vi "prompts get.vi"(8 "error in":errorcluster, 10 "id":i32, 11 "message json":string) -> (0 "error out":errorcluster, 3 "response":string)   [LabVIEW 2020, in "MCP Server.lvlib"]
uses:
  MCP Server.lvlib
  Output Parameter.ctl
  Input Parameter.ctl
  36169f03-25f9-42a4-b558-7da57aa14dd0.vi
  7d3bd472-2036-4192-96a4-2be547f36210.vi
  14c59c94-2525-420a-b2b2-c4c9036dcf4d.vi
  <vilib>/JDP Science/JSONtext/Next JSON Value.vi
  <vilib>/JDP Science/JSONtext/String Subset.vi
  <vilib>/JDP Science/JSONtext/Parsing/Advance past next JSON Value (inlined COPY).vi
  <vilib>/JDP Science/JSONtext/Parsing/Advance past whitespace.vi
  <vilib>/JDP Science/JSONtext/Parsing/Advance past String.vi
  <vilib>/JDP Science/JSONtext/Parsing/Advance past Number.vi
  <vilib>/JDP Science/JSONtext/Parsing/Advance past Line Ending.vi
  <vilib>/JDP Science/JSONtext/Parsing/Parse Full Path or Item Name.vi
  <vilib>/JDP Science/JSONtext/Parsing/Advance past Array.vi
  <vilib>/JDP Science/JSONtext/Parsing/Advance past Object.vi
  <vilib>/JDP Science/JSONtext/support/Error Cluster From Code.vi
  <vilib>/JDP Science/JSONtext/Offset/Find Item Locations by Path.vi
  <vilib>/JDP Science/JSONtext/JSON text to Variant.vi
  <vilib>/Utility/error.llb/Error Cluster From Error Code.vi
  <vilib>/JDP Science/JSONtext/Variant to JSON Text.vi
  <vilib>/JDP Science/JSONtext/support/Format JSON Object.vi
  <vilib>/JDP Science/JSONtext/support/Format JSON Array Text.vi
  <vilib>/JDP Science/JSONtext/LVClass Serializer/JSONtext LVClass Serializer.lvclass
  <vilib>/ErrorRing/Error Ring.xnode
  <vilib>/JDP Science/JSONtext/JSONtext.lvlib
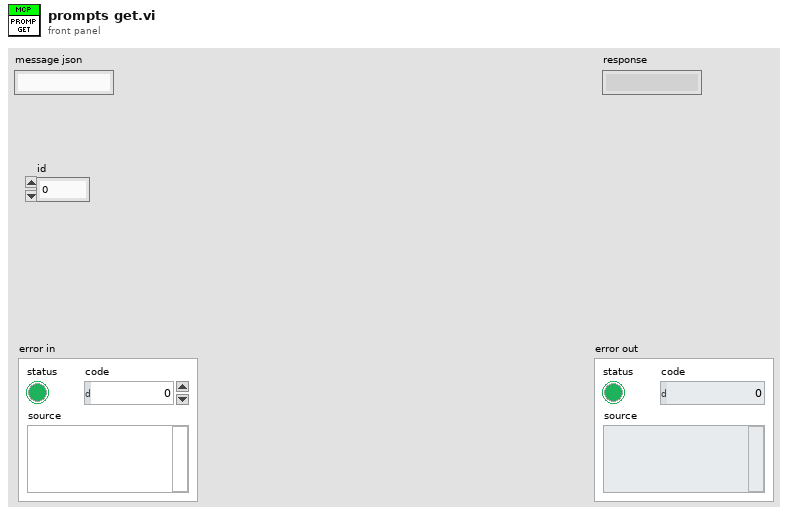
[diagram p1: front panel]
types:
  T1 = typedef "MCP Server.lvlib/Output Parameter.ctl" = cluster{"name":string, "description":string, "type":string, "raw name":string}
  T2 = typedef "MCP Server.lvlib/Prompt Data.ctl" = cluster{"name":string, "description":string, "arguments":T3[], "return terminal name":string, "results description":string, "VI Refnum":refnum<vi>}
  T3 = typedef "MCP Server.lvlib/Prompt Argument.ctl" = cluster{"name":string, "description":string, "required":bool, "raw_name":string}
  T4 = typedef "MCP Server.lvlib/Input Parameter.ctl" = cluster{"name":string, "type":string, "description":string, "required":bool, "raw name":string}
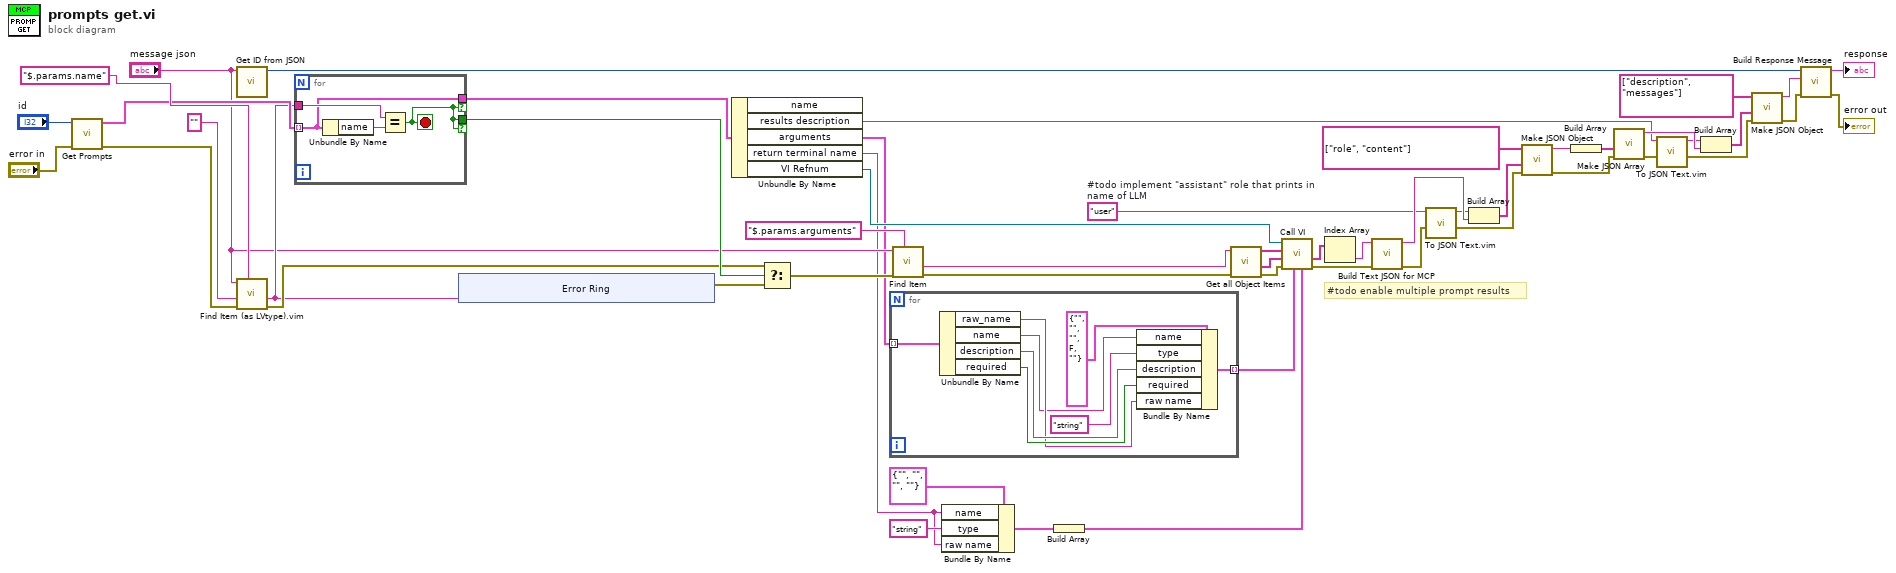
[diagram p0: block diagram]
diagram:
  w9 = "user"  # #todo implement "assistant" role that prints in name of LLM
  # "#todo enable multiple prompt results"
  n1 = call "Get Prompts.vi"("error in (no error)"="error in", "id"="id") -> ("error out"=w49:errorcluster, "Prompts"=w48:T2[])  [unwired: 8 in]
  n2 = call "Get ID from JSON.vi"("message json"="message json") -> ("Data out"=w2:i32)  [unwired: 10 in]
  n3 = call "Find Item (as LVtype).vim"("$Path or Item Name"="$.params.name", "error in (no error)"=w49, "Data Type and Default Value"="" ("$Path or Item Name"), "JSON"="message json") -> ("error out"=w43:errorcluster, "Data"=w41:string)  [unwired: 4 in, 2 out]
  n4 = for {
    tunnel: w41 -> [w55]
    tunnel: w48 -> [w54] mode=indexing
    tunnel: [w54] -> w44 if=w53
    tunnel: [w53] -> w45 if=w53
    stop <- w53 stop-if-true
    n5 = Unbundle By Name(w54) -> ("name"=w56:string)
    n6 = Equal?(x=w55, y=w56) -> (x = y?=w53:bool)
  }
  n7 = xnode "Error Ring"("parameter 0"=w41) -> ("error out"=w46:errorcluster)
  n8 = Unbundle By Name(w44) -> ("results description"=w6:string, "arguments"=w31:T3[], "return terminal name"=w11:string, "VI Refnum"=w32:refnum<vi>)  [unwired: 1 out]
  n9 = Select(t=w43, s=w45, f=w46) -> (s? t:f=w47:errorcluster)
  n10 = for {
    tunnel: w31 -> [w62] mode=indexing
    tunnel: [w63] -> w26 mode=indexing
    n11 = Unbundle By Name(w62) -> ("raw_name"=w58:string, "name"=w57:string, "description"=w61:string, "required"=w60:bool)
    n12 = Bundle By Name(cluster=T4 {"name"="", "type"="", "description"="", "required"=FALSE, "raw name"=""} ("Cluster"), "name"=w57, "type"="string", "description"=w61, "required"=w60, "raw name"=w58) -> (w63:T4)
  }
  n13 = call <vilib>:"Find Item.vi"("$Path or Item Name"="$.params.arguments", "error in (no error)"=w47, "JSON"="message json") -> ("error out"=w23:errorcluster, "<JSON>"=w25:string)  [unwired: 5 in, 2 out]
  n14 = Bundle By Name(cluster=T1 {"name"="", "description"="", "type"="", "raw name"=""} ("Cluster"), "name"=w11, "type"="string", "raw name"=w11) -> (w28:T1)
  n15 = Build Array(w28) -> (w29:T1[])
  n16 = call <vilib>:"Get all Object Items.vi"("error in (no error)"=w23, "JSON"=w25) -> ("error out"=w22:errorcluster, "<JSON>"=w24:string[], "Item Names"=w21:string[])  [unwired: 6 in, 1 out]
  n17 = call "Call VI.vi"("output info"=w29, "input info"=w26, "error in (no error)"=w22, "Input Values"=w24, "Input Names"=w21, "VI in"=w32) -> ("error out"=w33:errorcluster, "output values"=w16:string[])  [unwired: 2 in, 2 out]
  n18 = Index Array(array=w16) -> (element=w14:string)  [unwired: 1 in]
  n19 = call "Build Text JSON for MCP.vi"("error in (no error)"=w33, "text in"=w14) -> ("error out"=w15:errorcluster, "MCP JSON text content"=w13:string)  [unwired: 8 in]
  n20 = call "To JSON Text.vim"("error in (no error)"=w15, "Anything"=w9) -> ("error out"=w10:errorcluster, "<JSON>"=w8:string)  [unwired: 8 in]
  n21 = Build Array(w8, w13) -> (w18:string[])
  n22 = call <vilib>:"Make JSON Object.vi"("error in (no error)"=w10, "JSON Items"=w18, "Item Names"=string[] ["role", "content"]) -> ("error out"=w20:errorcluster, "<JSON>"=w17:string)  [unwired: 7 in]
  n23 = Build Array(w17) -> (w12:string[])
  n24 = call <vilib>:"Make JSON Array.vi"("error in (no error)"=w20, "JSON Elements"=w12) -> ("error out"=w38:errorcluster, "<JSON>"=w34:string)  [unwired: 8 in]
  n25 = call "To JSON Text.vim"("error in (no error)"=w38, "Anything"=w6) -> ("error out"=w7:errorcluster, "<JSON>"=w5:string)  [unwired: 8 in]
  n26 = Build Array(w5, w34) -> (w35:string[])
  n27 = call <vilib>:"Make JSON Object.vi"("error in (no error)"=w7, "JSON Items"=w35, "Item Names"=string[] ["description", "messages"]) -> ("error out"=w37:errorcluster, "<JSON>"=w1:string)  [unwired: 7 in]
  n28 = call "Build Response Message.vi"("error in (no error)"=w37, "Result content"=w1, "message id in"=w2) -> ("error out"=→"error out":errorcluster, "MCP message out"=→"response":string)  [unwired: 7 in]
